vi "Manual VMO.vi"(0 "System no.":i32=1 min=1 max=4 step=1, 2 "Axes to command":string[](array[string]), 3 "Position values":dbl[](array[numeric]) format="%.6f", 5 "error in":errorcluster, 6 "Minimum pos.":dbl[](array[numeric]) format="%.6f", 7 "Maximum pos.":dbl[](array[numeric]) format="%.6f") -> (14 "Move possible":bool, 19 "error out":errorcluster)   [LabVIEW 2026]
doc: "Virtual movement. Indicates whether a move to the specified position is possible or not by checking if the commanded position value is within the given position range. Stage will not be moved."
panel:
  # "Virtual movement. Indicates whether a move to the specified position is possible or not by checking\nif the commanded position value is within the given position range. Axes will NOT be moved."
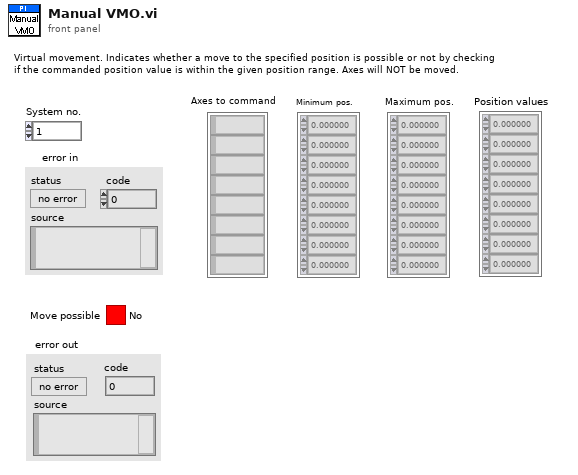
[diagram p1: front panel]
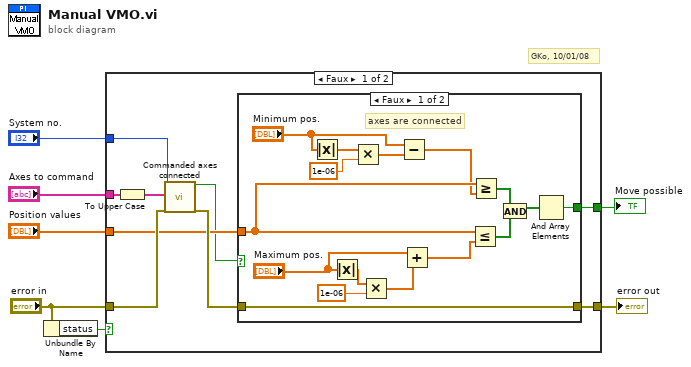
[diagram p0: block diagram]
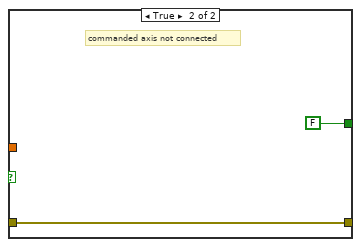
[diagram p2: hidden frame]
diagram:
  # "GKo, 10/01/08"
  n1 = Unbundle By Name("error in") -> ("status"=w1:bool)
  n2 = case shown="Faux" w1 {
    tunnel: [w16 w36] -> w7
    tunnel: "Position values" -> [w9 _]
    tunnel: "error in" -> [w15 w36]
    tunnel: "System no." -> [w10 _]
    tunnel: [w13 FALSE] -> w4
    tunnel: "Axes to command" -> [w12 _]
    frame False {
      n3 = To Upper Case(1:w12) -> (0:w11:string[])
      n4 = call "Commanded axes connected.vi"("System no."=w10, "Commanded axes"=w11, "error in"=w15) -> ("Controller error"=w8:bool, "error out"=w14:errorcluster)  [unwired: 1 in, 14 out]
      n5 = case shown="Faux" w8 {
        tunnel: [w32 w34] -> w16
        tunnel: w14 -> [w32 w34]
        tunnel: [w27 FALSE] -> w13
        tunnel: w9 -> [w31 _]
        frame False {
          # "axes are connected"
          n6 = Absolute Value(x="Minimum pos.") -> (abs(x)=w18:dbl[])
          n7 = Absolute Value(x="Maximum pos.") -> (abs(x)=w17:dbl[])
          n8 = Multiply(x=w18, y=1e-06 ("Numeric")) -> (x*y=w25:dbl[])
          n9 = Multiply(x=w17, y=1e-06 ("Numeric")) -> (x*y=w20:dbl[])
          n10 = Subtract(x="Minimum pos.", y=w25) -> (x-y=w23:dbl[])
          n11 = Add(x="Maximum pos.", y=w20) -> (x+y=w19:dbl[])
          n12 = Less Or Equal?(x=w31, y=w19) -> (x <= y?=w29:bool[])
          n13 = Greater Or Equal?(x=w31, y=w23) -> (x >= y?=w30:bool[])
          n14 = And(x=w30, y=w29) -> (x .and. y?=w28:bool[])
          n15 = And Array Elements(Boolean array=w28) -> (logical AND=w27:bool)
        }
        frame True {
          # "commanded axis not connected"
        }
      }
    }
    frame True {
    }
  }
  "error out" <- w7
  "Move possible" <- w4
